vi "ReadVoltage_DDR.vi"(6 "error in (no error)":errorcluster, 9 "Voltage to Measure":string(combo)="Bandgap") -> (0 "error out":errorcluster, 3 "Voltage Read":dbl)   [LabVIEW 2011]
doc: "This VI reads a chosen voltage of a DDR PLL.\n\nInputs:\n1. Voltage to Measure: Selects the voltage that will be read by the SRP ADC (ie. BG, VA, VD, etc.).\n\nOutputs:\n1.Voltage Read: The value of the chosen measurement in volts."
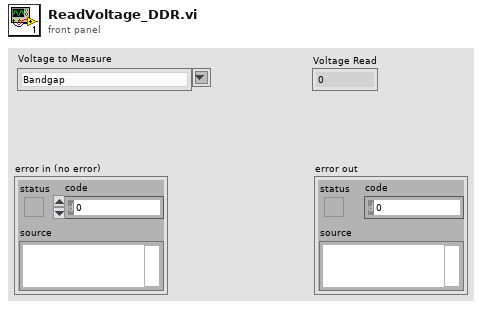
[diagram p1: front panel]
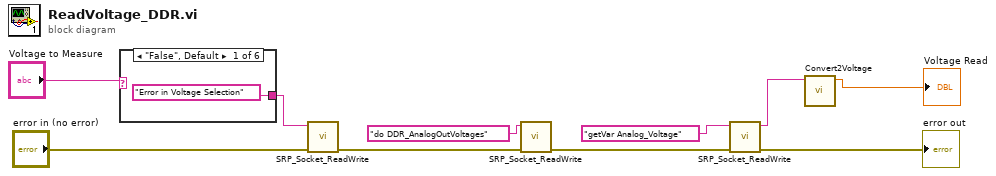
[diagram p0: block diagram]
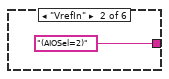
[diagram p2: hidden frame]
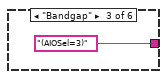
[diagram p3: hidden frame]
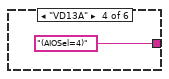
[diagram p4: hidden frame]
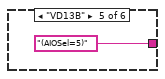
[diagram p5: hidden frame]
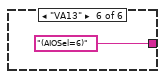
[diagram p6: hidden frame]
diagram:
  n1 = case shown="\"False\", Default" "Voltage to Measure" {
    tunnel: ["Error in Voltage Selection" "(AIOSel=2)" "(AIOSel=3)" "(AIOSel=4)" "(AIOSel=5)" "(AIOSel=6)"] -> w5
    frame "False", Default {
    }
    frame "VrefIn" {
    }
    frame "Bandgap" {
    }
    frame "VD13A" {
    }
    frame "VD13B" {
    }
    frame "VA13" {
    }
  }
  n2 = call "SRP_Socket_ReadWrite.vi"("error in (no error)"="error in (no error)", "Data In"=w5) -> ("error out"=w7:errorcluster)  [unwired: 7 in, 1 out]
  n3 = call "SRP_Socket_ReadWrite.vi"("error in (no error)"=w7, "Data In"="do DDR_AnalogOutVoltages") -> ("error out"=w8:errorcluster)  [unwired: 7 in, 1 out]
  n4 = call "SRP_Socket_ReadWrite.vi"("error in (no error)"=w8, "Data In"="getVar Analog_Voltage") -> ("error out"=→"error out":errorcluster, "Data Out"=w2:string)  [unwired: 7 in]
  n5 = call "Convert2Voltage.vi"("SRP ADC String"=w2) -> ("Voltage"=→"Voltage Read":dbl)  [unwired: 10 in]
